vi "FGV_PeriodicTasks.vi"(0 "MIDAS Commands":T1, 4 "Task":enum16{"AddTask", "GetTasks", "ClearTasks"}(ring)) -> (5 "Tasks":string[](array[string]))   [LabVIEW 2018, in "feGEM DataPacker.lvlib"]
uses:
  feGEM DataPacker.lvlib
  Utilities/PeriodicEnumTypeDef.ctl
  <vilib>/Utility/SystemLogging/NI_SystemLogging.lvlib
panel:
  in  "Task List":T1
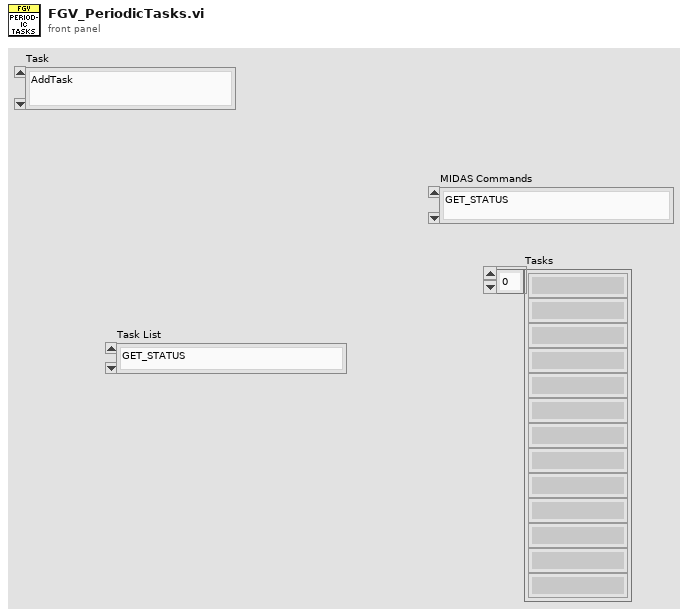
[diagram p1: front panel]
types:
  T1 = typedef "feGEM DataPacker.lvlib/PeriodicEnumTypeDef.ctl" = enum16{"GET_STATUS", "GET_HIST_RATE", "GET_RUNNO", "GET_RUN_START_T", "GET_RUN_STOP_T", "GET_TIME", "ENABLE_DEBUG_MODE"}
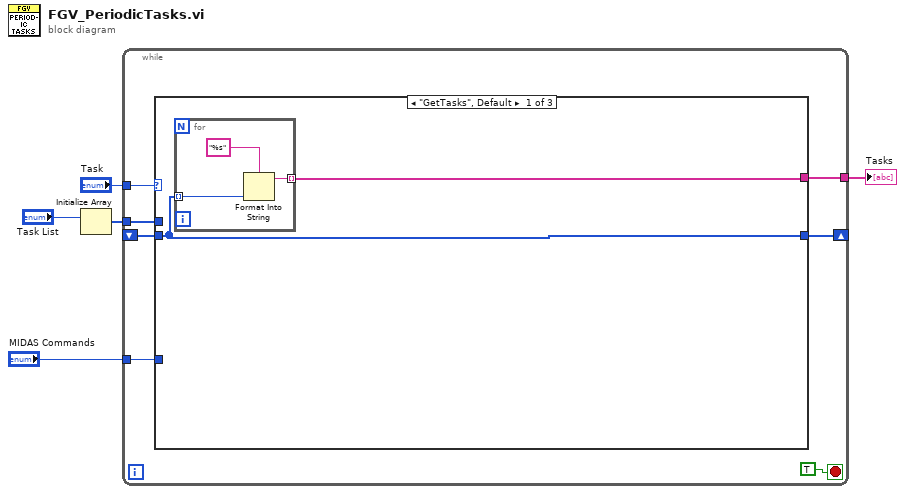
[diagram p0: block diagram]
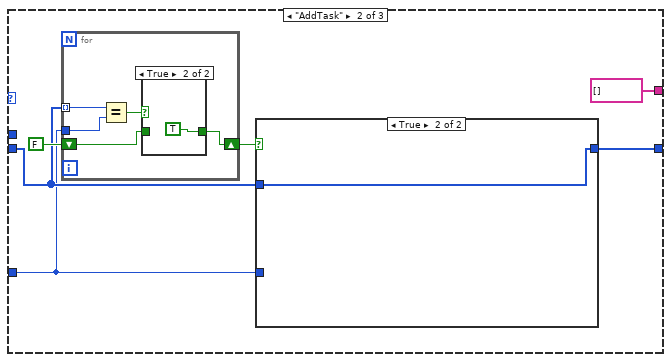
[diagram p2: hidden frame]
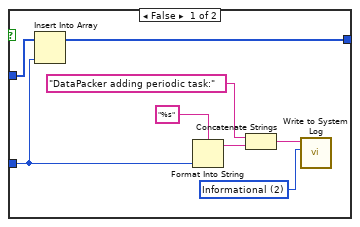
[diagram p3: hidden frame]
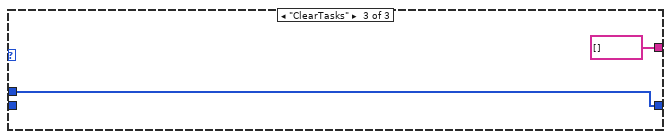
[diagram p5: hidden frame]
diagram:
  n1 = Initialize Array("Task List") -> (w1:T1[])  [unwired: 1 in]
  n2 = while {
    shift-right: [w11] -> _
    shift-left: _ -> [w12]
    tunnel: "MIDAS Commands" -> [w9]
    tunnel: "Task" -> [w8]
    tunnel: [w7] -> w3
    tunnel: w1 -> [w6]
    stop <- TRUE stop-if-true
    n3 = case shown="\"GetTasks\", Default" w8 {
      tunnel: [w13 w21 w41] -> w11
      tunnel: w12 -> [w13 w20 _]
      tunnel: w9 -> [_ w18 _]
      tunnel: [w14 string[] [] string[] []] -> w7
      tunnel: w6 -> [_ _ w41]
      frame "GetTasks", Default {
        n4 = for {
          tunnel: [w16] -> w14 mode=indexing
          tunnel: w13 -> [w15] mode=indexing
          n5 = Format Into String(format string="%s" ("string (\"\")"), w15) -> (resulting string=w16:string)  [unwired: 2 in, 1 out]
        }
      }
      frame "AddTask" {
        n6 = for {
          tunnel: w20 -> [w37] mode=indexing
          shift-right: [w35] -> w22
          shift-left: FALSE -> [w34]
          tunnel: w18 -> [w33]
          n7 = Equal?(x=w37, y=w33) -> (x = y?=w36:bool)
          n8 = case shown="True" w36 {
            tunnel: [w38 TRUE] -> w35
            tunnel: w34 -> [w38 _]
            frame False {
            }
            frame True {
            }
          }
        }
        n9 = case shown="True" w22 {
          tunnel: w20 -> [w31 w32]
          tunnel: [w30 w32] -> w21
          tunnel: w18 -> [w25 _]
          frame False {
            w27 = 2 items=["Error", "Warning", "Informational"] ("severity")
            n10 = Insert Into Array(array=w31, new element=w25) -> (w30:T1[])  [unwired: 1 in]
            n11 = Format Into String(format string="%s" ("string (\"\")"), w25) -> (resulting string=w29:string)  [unwired: 2 in, 1 out]
            n12 = Concatenate Strings("DataPacker adding periodic task:" ("string"), w29) -> (w24:string)
            n13 = call <vilib>:"Write to System Log.vi"("severity"=w27, "message"=w24) -> ()  [unwired: 9 in, 1 out]
          }
          frame True {
          }
        }
      }
      frame "ClearTasks" {
      }
    }
  }
  "Tasks" <- w3
